vi "algoritmo_6.vi"() -> ()   [LabVIEW 2024]
uses:
  <vilib>/Platform/TimedLoop/XDataNode/timing_clust.ctl
  <vilib>/Platform/TimedLoop/XDataNode/nitl_modes.ctl
  <vilib>/Platform/TimedLoop/XDataNode/wakeup.ctl
  <vilib>/MakerHub/LINX/Public/Peripherals/PWM/PWM Set Duty Cycle 1 Chan.vi
  <vilib>/MakerHub/LINX/Public/Utilities/Open Serial.vi
  <vilib>/MakerHub/LINX/Public/Peripherals/PWM/PWM Set Duty Cycle N Chans.vi
  <vilib>/platform/TimedLoop/XDataNode/XDataNode.xnode
  <vilib>/Platform/TimedLoop/XDataNode/XDNodeRunTimeDep.lvlib
  <vilib>/MakerHub/LINX/LMH-LINX.lvlib
  <vilib>/MakerHub/LINX/Public/Sensors/Distance/Ultrasonic/Ultrasonic.lvlib
  <vilib>/Analysis/NI_AALPro.lvlib
panel:
  out "error":dbl
  out "POLO":dbl
  in  "Slide":dbl(slide) scale=0.5..0.65
  in  "Numeric":dbl
  in  "Referencia 2":dbl(slide) scale=-41.0..41.0
  out "Error":dbl
  out "PWM":dbl format="%0.2f"
  out "xk1":dbl[](array[numeric])
  out "uk":dbl
  in  "Referencia":dbl(slide) scale=5.0..41.0
  out "ESTADO":dbl
  out "MINUTOS":dbl format="%#_2g"
  out "y_estimada":dbl
  out "error de estimacion":dbl
  out "THETA":cdb[](array[numeric])
  out "Waveform Chart":T1(graph)
  in  "stop":bool
  in  "Serial Port":refnum<visa-resource-name>="N/A"
  out "Error Out":errorcluster
  out "Y_Real":fxp<+/-,64,32>
  # "1 PARA ESTIMAR"
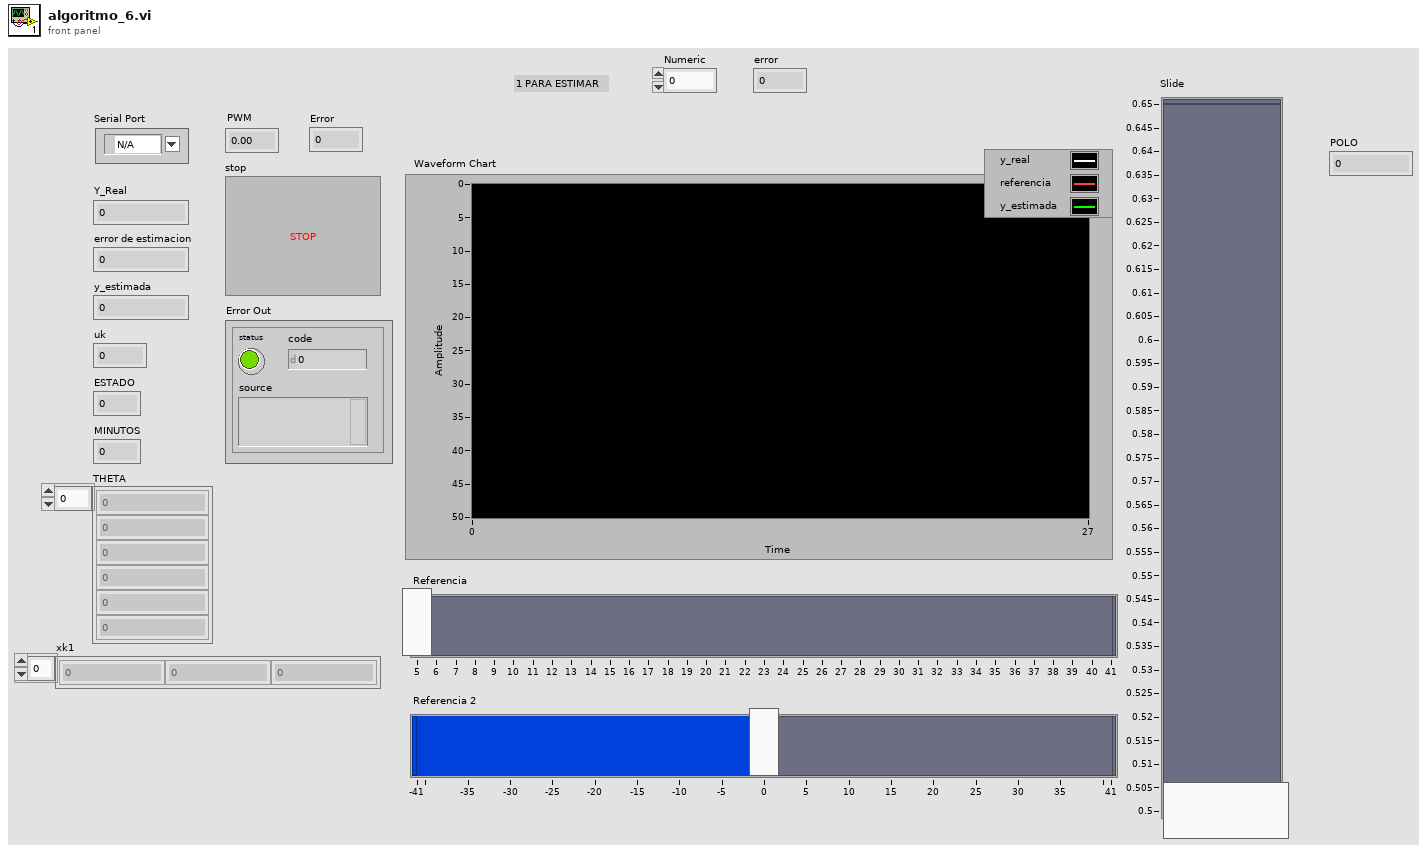
[diagram p1: front panel]
types:
  T1 = cluster{"Centimeters":dbl, "Referencia":dbl, dbl}
  T2 = typedef "LMH-LINX.lvlib/LINX Ref.ctl" = cluster{"IO":T3, "Interface":T4, "LINX Device Config":T5}
  T3 = typedef "LMH-LINX.lvlib/Platform.ctl" = enum16{"Remote", "Local"}
  T4 = typedef "LMH-LINX.lvlib/Interface.ctl" = enum16{"Serial", "TCP"}
  T5 = typedef "LMH-LINX.lvlib/Device.lvlib/LINX Device Config.ctl" = cluster{"Interface":T4, "COM Port":refnum<visa-resource-name>, "TCP Configuration":T6, "Device Family":u8, "Device ID":u8, "Device Name":string, "TCP Ref":refnum<k5>, "Channels":T7}
  T6 = typedef "LMH-LINX.lvlib/Device.lvlib/TCP Config.ctl" = cluster{"IP Address":string, "Port":u16}
  T7 = typedef "LMH-LINX.lvlib/Channels.ctl" = cluster{"DI":u8[], "DO":u8[], "AI":u8[], "AO":u8[], "PWM":u8[], "QE":u8[], "UART":u8[], "I2C 2":u8[], "SPI":u8[], "CAN":u8[], "Servo":u8[], "AI Ref (V)":dbl, "AI Resolution (Bits)":u8, "AO Ref (V)":dbl, "AO Resolution (Bits)":u8}
  T8 = typedef "XDNodeRunTimeDep.lvlib/timing_clust.ctl" = cluster{"Expected End [f-1]":u64, "Actual End [f-1]":u64, "Finished Late? [f-1]":bool, "Expected End [i-1]":u64, "Actual End [i-1]":u64, "Finished Late? [i-1]":bool, "Expected Start [i]":u64, "Actual Start [i]":u64, "Expected Start [f]":u64, "Actual Start [f]":u64, "Source Name":string, "Structure Name":string, "Period":i64, "Deadline":i64, "Offset":i64, "Start":i64, "Priority":i32, "Timeout":i32, "Mode":T9, "Wakeup Reason":T10, "Error":errorcluster, "Source Type":string, "Secondary Source Type":string, "Global End Time":u64, "Global Start Time":u64, "Frame Duration":u64, "Iteration Duration":u64, "Assigned CPU":i32, "I/O Scan Engine Mode":u32}
  T9 = typedef "XDNodeRunTimeDep.lvlib/nitl_modes.ctl" = enum32{"No Change", "Process missed periods, maintain original phase", "Discard missed periods, maintain original phase", "Process missed periods, ignore original phase", "Discard missed periods, ignore original phase"}
  T10 = typedef "XDNodeRunTimeDep.lvlib/wakeup.ctl" = enum32{"Normal", "Aborted", "Asynchronous wakeup", "Timing source error", "Timed loop error", "Timeout"}
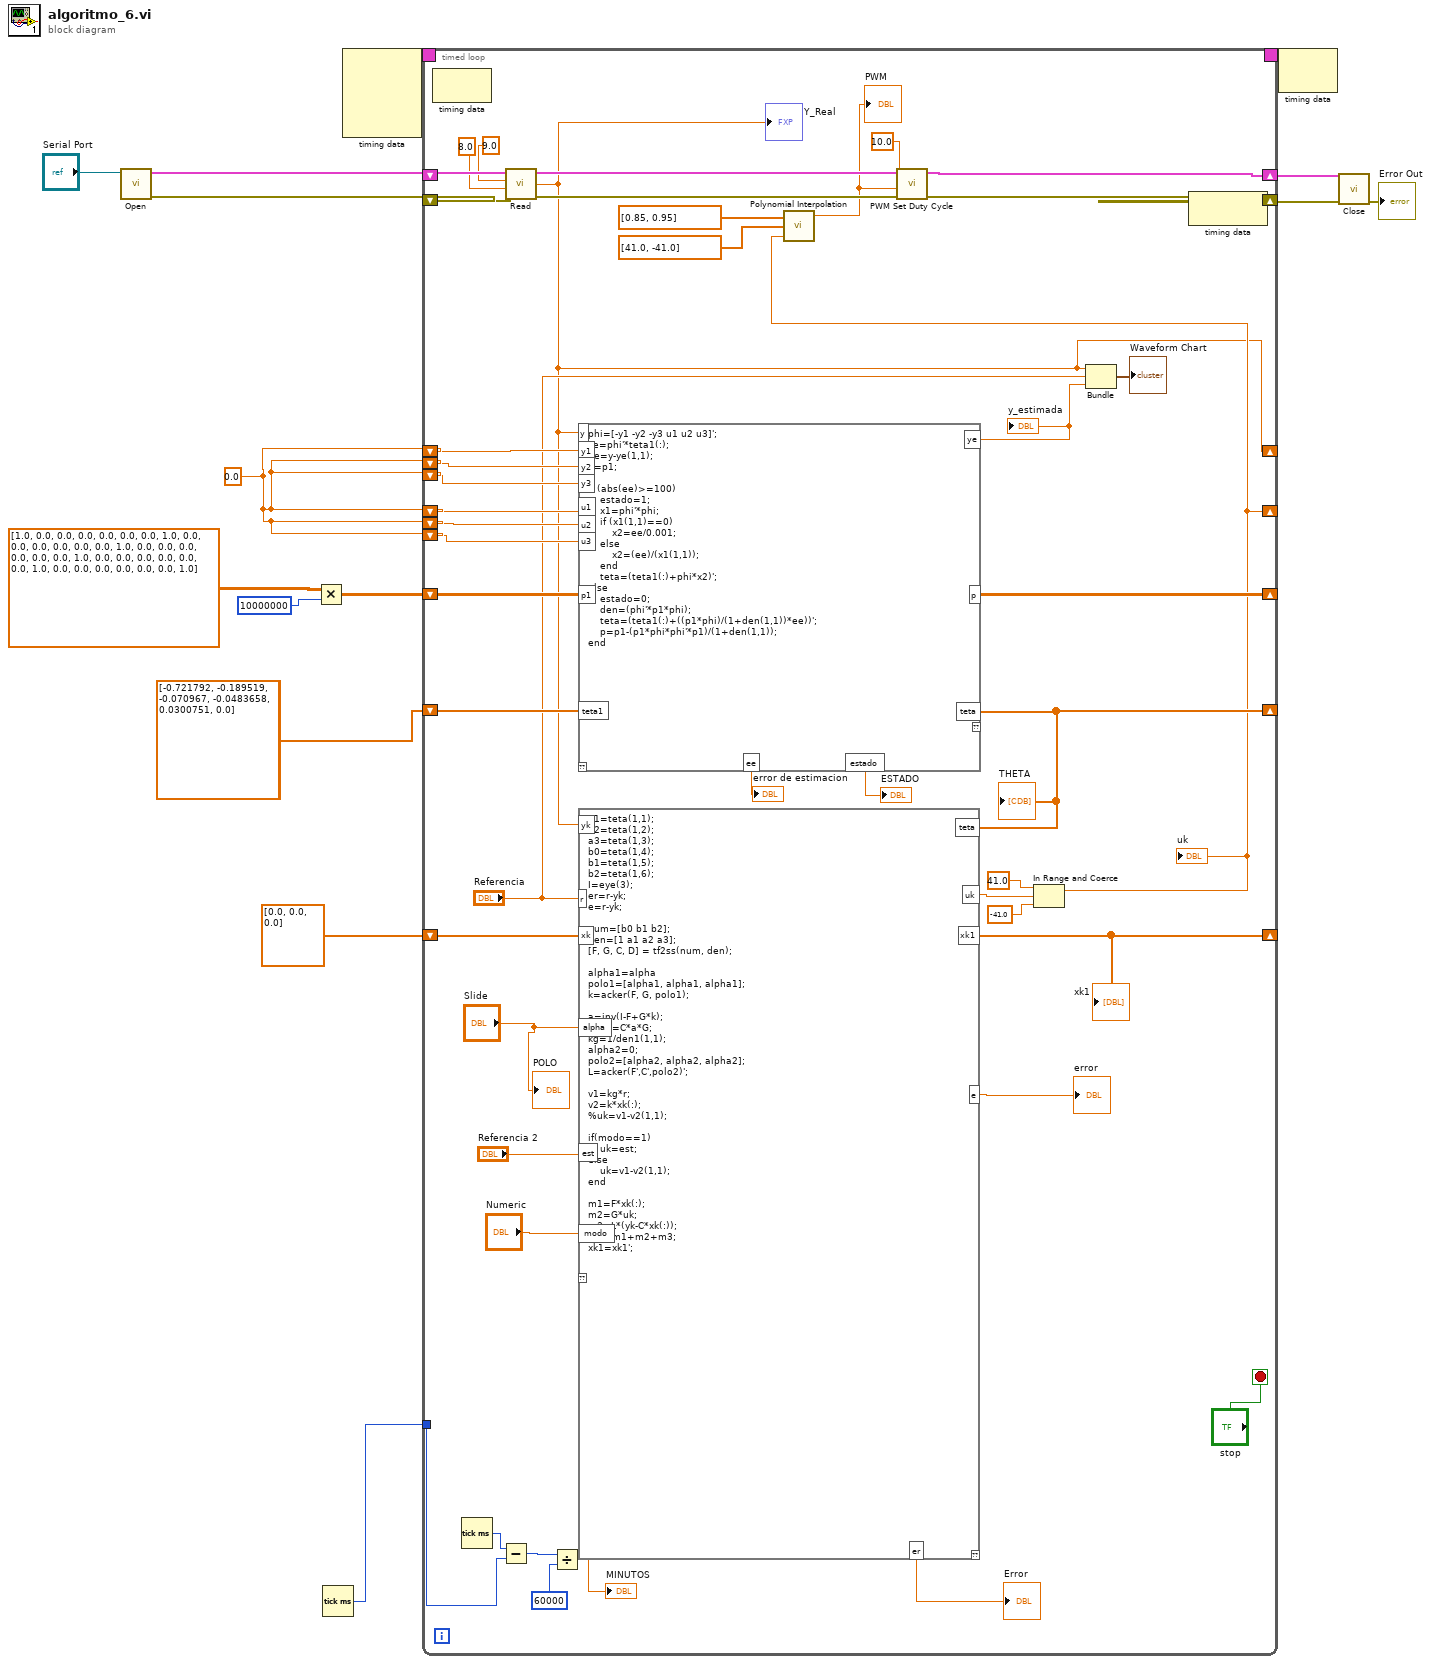
[diagram p0: block diagram]
diagram:
  (unwired) dbl[] [-0.721792, -0.189519, -0.070967, -0.0483658, 0.0300751, 0.0]
  w7 = 0.0
  n1 = call-poly <vilib>:"Open.vi"("Serial Port"="Serial Port") -> ("Error Out"=w11:errorcluster, "LINX Resource"=w13:T2)  [unwired: 8 in, 1 out]
  n2 = Multiply(x=dbl[][] [[1.0, 0.0, 0.0, 0.0, 0.0, 0.0], [0.0, 1.0, 0.0, 0.0, 0.0, 0.0], [0.0, 0.0, 1.0, 0.0, 0.0, 0.0], [0.0, 0.0, 0.0, 1.0, 0.0, 0.0], [0.0, 0.0, 0.0, 0.0, 1.0, 0.0], [0.0, 0.0, 0.0, 0.0, 0.0, 1.0]], y=10000000) -> (x*y=w4:dbl[][])
  n3 = Tick Count (ms)() -> (millisecond timer value=w3:u32)
  n4 = node-c288() -> (w15:T8)  [unwired: 4 in]
  n5 = timed-loop {
    timing: w15 -> [_]
    timing-out: [_] -> w14
    shift-right: [w48] -> w12
    shift-left: w13 -> [w60]
    shift-right: [w54] -> w10
    shift-left: w11 -> [w59]
    shift-right: [w29] -> _
    shift-left: dbl[] [-0.935317, -0.055731, -0.0173078, -0.00504643, 0.00837056, 0.00547238] -> [w47]
    shift-right: [w20] -> _
    shift-left: w7 -> [w45]
    shift-right: [w22] -> _
    shift-left: w7 -> [w46]
    shift-left: w7 -> [w44]
    shift-left: w7 -> [w43]
    shift-left: w7 -> [w42]
    shift-left: w7 -> [w41]
    shift-right: [w38] -> _
    shift-left: w4 -> [w39]
    tunnel: w3 -> [w34]
    shift-right: [w28] -> _
    shift-left: dbl[] [0.0, 0.0, 0.0] -> [w27]
    stop <- "stop" stop-if-true
    n6 = node-c288() -> ()  [unwired: 1 in, 1 out]
    n7 = Tick Count (ms)() -> (millisecond timer value=w35:u32)
    n8 = Subtract(x=w35, y=w34) -> (x-y=w32:u32)
    n9 = call <vilib>:"Read.vi"("Error In"=w59, "DO Channel"=8.0, "DI Channel"=9.0, "LINX Resource"=w60) -> ("Error Out"=w55:errorcluster, "Centimeters"=w20:dbl, "LINX Resource"=w56:T2)  [unwired: 4 in, 1 out]
    "Y_Real" <- w20
    n10 = Divide(x=w32, y=u32 60000) -> (x/y=→"MINUTOS":dbl)
    n11 = script code="phi=[-y1 -y2 -y3 u1 u2 u3]';\nye=phi'*teta1(:);\nee=y-ye(1,1);\np=p1;\n\nif (abs(ee)>=100)\n    estado=1;\n    x1=phi'*phi;\n    if (x1(1,1)==0)\n        x2=ee/0.001;\n    else\n        x2=(ee)/(x1(1,1));\n    end\n    teta=(teta1(:)+phi*x2)';\nelse\n    estado=0;\n    den=(phi'*p1*phi);\n    teta=(teta1(:)+((p1*phi)/(1+den(1,1))*ee))';\n    p=p1-(p1*phi*phi'*p1)/(1+den(1,1));\nend"("teta1"=w47, "y1"=w45, "y2"=w44, "y3"=w43, "u1"=w46, "u2"=w42, "u3"=w41, "y"=w20, "p1"=w39) -> ("teta"=w29:dbl[], "p"=w38:dbl[][], "ye"=w37:dbl, "ee"=→"error de estimacion":dbl, "estado"=→"ESTADO":dbl)  [unwired: 1 in, 1 out]
    "THETA" <- w29
    "y_estimada" <- w37
    n12 = script code="a1=teta(1,1);\na2=teta(1,2);\na3=teta(1,3);\nb0=teta(1,4);\nb1=teta(1,5);\nb2=teta(1,6);\nI=eye(3);\ner=r-yk;\ne=r-yk;\n\nnum=[b0 b1 b2];\nden=[1 a1 a2 a3];\n[F, G, C, D] = tf2ss(num, den);\n\nalpha1=alpha\npolo1=[alpha1, alpha1, alpha1]; \nk=acker(F, G, polo1);\n\na=inv(I-F+G*k);\nden1=C*a*G;\nkg=1/den1(1,1);\nalpha2=0;\npolo2=[alpha2, alpha2, alpha2]; \nL=acker(F',C',polo2)';\n\nv1=kg*r;\nv2=k*xk(:);\n%uk=v1-v2(1,1);\n\nif(modo==1)\n    uk=est;\nelse\n    uk=v1-v2(1,1);\nend\n\nm1=F*xk(:);\nm2=G*uk;\nm3=L*(yk-C*xk(:));\nxk1=m1+m2+m3;\nxk1=xk1';"("teta"=w29, "xk"=w27, "yk"=w20, "r"="Referencia", "alpha"="Slide", "est"="Referencia 2", "modo"="Numeric") -> ("xk1"=w28:dbl[], "uk"=w23:dbl, "er"=→"Error":dbl, "e"=→"error":dbl)  [unwired: 1 in, 1 out]
    "xk1" <- w28
    n13 = In Range and Coerce(upper limit=41.0, x=w23, lower limit=-41.0) -> (coerced(x)=w22:dbl)  [unwired: 1 out]
    "uk" <- w22
    n14 = call <vilib>:"Polynomial Interpolation.vi"("x value"=w22, "X"=dbl[] [41.0, -41.0], "Y"=dbl[] [0.85, 0.95]) -> ("interpolation value"=w50:dbl)  [unwired: 2 out]
    "PWM" <- w50
    n15 = call-poly <vilib>:"PWM Set Duty Cycle.vi"("Error In"=w55, "Duty Cycle (0-1)"=w50, "PWM Channel"=10.0, "LINX Resource"=w56) -> ("Error Out"=w54:errorcluster, "LINX Resource"=w48:T2)  [unwired: 6 in]
    n16 = Bundle("Centimeters"=w20, "Referencia"="Referencia", w37) -> (→"Waveform Chart":T1)  [unwired: 1 in]
    n17 = node-c288() -> ()  [unwired: 1 in, 1 out]
    "POLO" <- "Slide"
  }
  n18 = node-c288(w14) -> ()  [unwired: 1 out]
  n19 = call <vilib>:"Close.vi"("Error In"=w10, "LINX Resource"=w12) -> ("Error Out"=→"Error Out":errorcluster)  [unwired: 9 in]
